vi "CALC_Calculate_phi_theta_etc_2_(offline).vi"(0 "Input data cluster":T2, 1 "SB size":u8, 5 "Twisted neck":bool, 7 "Bridge swap":bool, 9 "Use alternative magnets orientation":bool, 11 "Error In":errorcluster) -> (4 "Animal coordinates cluster":T1, 15 "Error out":errorcluster)   [LabVIEW 2018, in "Tracker.lvlib"]
uses:
  Tracker.lvlib
  Controls/CTL_Cage_Coords_(arrays).ctl
  Controls/CTL_Animal_Coordinates_and_Speed_(arr).ctl
  Controls/CTL_Animal_Coordinates_and_Speed.ctl
  <vilib>/ptbypt/NI_PtbyPt.lvlib
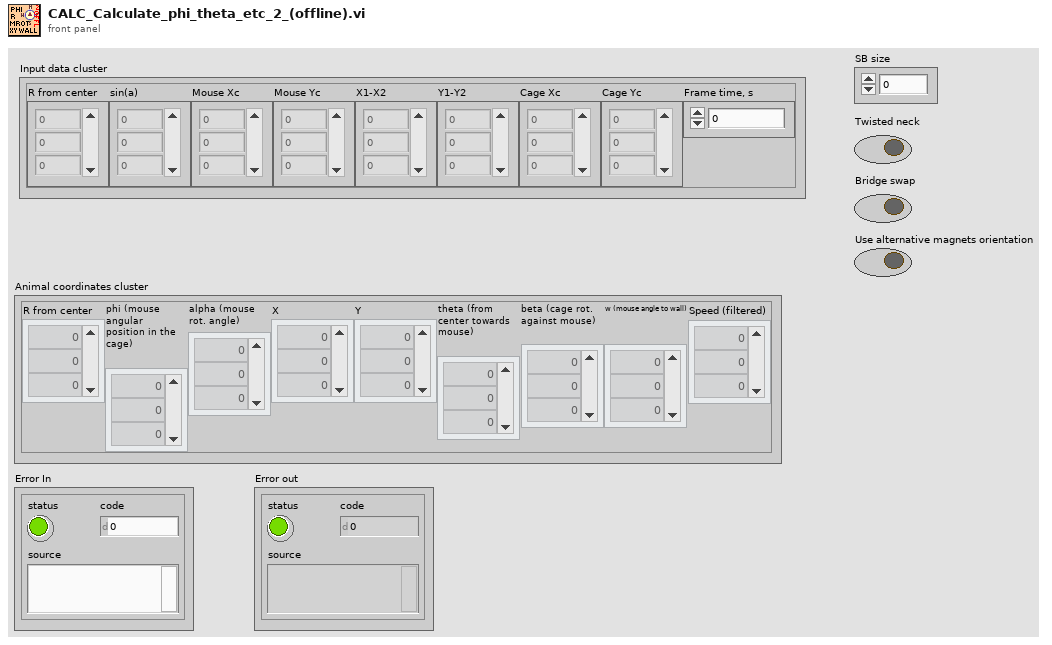
[diagram p1: front panel]
types:
  T1 = typedef "Tracker.lvlib/CTL_Animal_Coordinates_and_Speed_(arr).ctl" = cluster{"R from center":dbl[], "phi (mouse angular position in the cage)":dbl[], "alpha (mouse rot. angle)":dbl[], "X":dbl[], "Y":dbl[], "theta (from center towards mouse)":dbl[], "beta (cage rot. against mouse)":dbl[], "w (mouse angle to wall)":dbl[], "Speed (filtered)":dbl[]}
  T2 = typedef "Tracker.lvlib/CTL_Cage_Coords_(arrays).ctl" = cluster{"R from center":dbl[], "sin(a)":dbl[], "Mouse Xc":dbl[], "Mouse Yc":dbl[], "X1-X2":dbl[], "Y1-Y2":dbl[], "Cage Xc":dbl[], "Cage Yc":dbl[], "Frame time, s":dbl}
  T3 = typedef "Tracker.lvlib/CTL_Animal_Coordinates_and_Speed.ctl" = cluster{"R from center":dbl, "phi (mouse angular position in the cage)":dbl, "alpha (mouse rot. angle)":dbl, "X":dbl, "Y":dbl, "theta (from center towards mouse)":dbl, "beta (cage rot. against mouse)":dbl, "w (mouse angle to wall)":dbl, "Speed (filtered)":dbl}
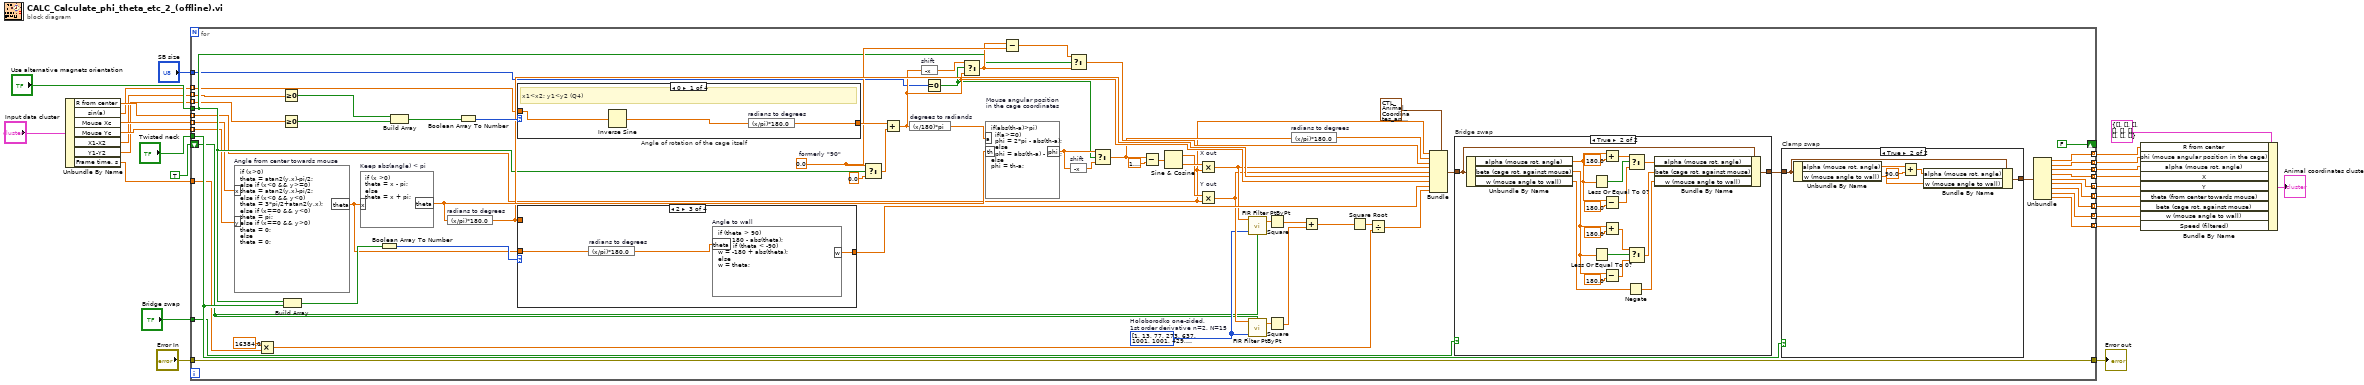
[diagram p0: block diagram]
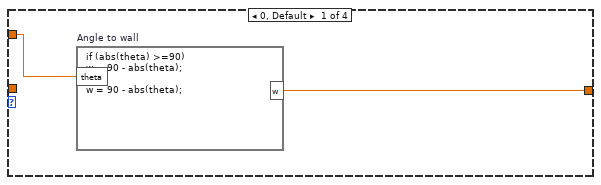
[diagram p3: hidden frame]
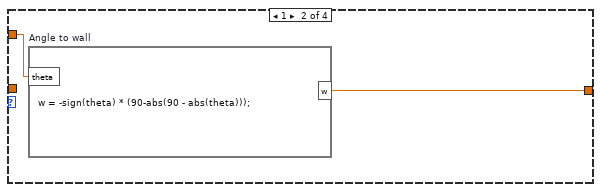
[diagram p4: hidden frame]
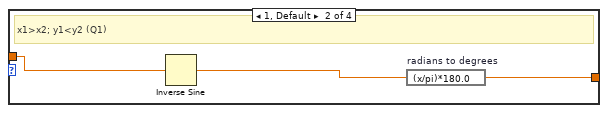
[diagram p7: hidden frame]
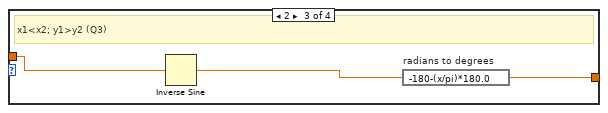
[diagram p8: hidden frame]
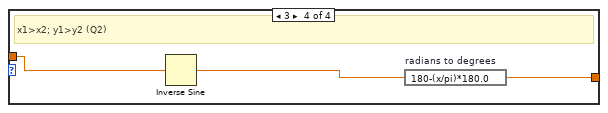
[diagram p9: hidden frame]
diagram:
  n1 = Unbundle By Name("Input data cluster") -> ("R from center"=w22:dbl[], "sin(a)"=w21:dbl[], "Mouse Xc"=w20:dbl[], "Mouse Yc"=w19:dbl[], "X1-X2"=w18:dbl[], "Y1-Y2"=w17:dbl[], "Frame time, s"=w16:dbl)
  n2 = for {
    tunnel: "Use alternative magnets orientation" -> [w67]
    tunnel: "Twisted neck" -> [w66]
    tunnel: "SB size" -> [w62]
    tunnel: "Bridge swap" -> [w48]
    tunnel: w22 -> [w47] mode=indexing
    tunnel: w21 -> [w46] mode=indexing
    tunnel: w20 -> [w45] mode=indexing
    tunnel: w19 -> [w44] mode=indexing
    tunnel: w18 -> [w43] mode=indexing
    tunnel: w17 -> [w42] mode=indexing
    tunnel: w16 -> [w41]
    tunnel: [w39] -> w13 mode=indexing
    tunnel: [w38] -> w12 mode=indexing
    tunnel: [w37] -> w11 mode=indexing
    tunnel: [w36] -> w10 mode=indexing
    tunnel: [w35] -> w9 mode=indexing
    tunnel: [w34] -> w8 mode=indexing
    tunnel: [w33] -> w7 mode=indexing
    tunnel: [w32] -> w6 mode=indexing
    tunnel: [w31] -> w5 mode=indexing
    tunnel: "Error In" -> [w30]
    tunnel: [w30] -> w2
    shift-right: [FALSE] -> _
    shift-left: TRUE -> [w29]
    w58 = i32[] [1, 13, 77, 273, 637, 1001, 1001, 429, -429, -1001, -1001, -637, -273, -77, -13, -1]  # Holoborodko one-sided, 1st order derivative n=2, N=15
    w77 = 0.0  # formerly "90"
    n3 = formula code="if (x>0)\ntheta = atan2(y,x)-pi/2;\nelse if (x<0 && y>=0)\ntheta = atan2(y,x)-pi/2;\nelse if (x<0 && y<0)\ntheta = 3*pi/2+atan2(y,x);\nelse if (x==0 && y<0)\ntheta = pi;\nelse if (x==0 && y>0)\ntheta = 0;\nelse\ntheta = 0;" "Angle from center towards mouse"("x"=w45, "y"=w44) -> ("theta"=w63:dbl)
    n4 = Multiply(x=16384.0 ("y"), y=w41) -> (x*y=w49:dbl)
    n5 = Greater Or Equal To 0?(x=w43) -> (x >= 0?=w94:bool)
    n6 = Greater Or Equal To 0?(x=w42) -> (x >= 0?=w93:bool)
    n7 = Build Array(w67, w66) -> (w65:bool[])
    n8 = formula code="if (x >0)\ntheta = x - pi;\nelse\ntheta = x + pi;" "Keep abs(angle) < pi"("x"=w63) -> ("theta"=w88:dbl)
    n9 = Boolean Array To Number(Boolean array=w65) -> (number=w64:u32)
    n10 = Build Array(w94, w93) -> (w92:bool[])
    n11 = expression code="(x/pi)*180.0" "radians to degrees"(w88) -> (w84:dbl)
    n12 = Boolean Array To Number(Boolean array=w92) -> (number=w91:u32)
    n13 = case "Angle of rotation of the cage itself" shown="0" w91 {
      tunnel: w46 -> [w130 w133 w136 w139]
      tunnel: [w129 w132 w135 w138] -> w80
      frame 0 {
        # "x1<x2; y1<y2 (Q4)"
        n14 = Inverse Sine(1:w130) -> (0:w131:dbl)
        n15 = expression code="(x/pi)*180.0" "radians to degrees"(w131) -> (w129:dbl)
      }
      frame 1, Default {
        # "x1>x2; y1<y2 (Q1)"
        n16 = Inverse Sine(1:w133) -> (0:w134:dbl)
        n17 = expression code="(x/pi)*180.0" "radians to degrees"(w134) -> (w132:dbl)
      }
      frame 2 {
        # "x1<x2; y1>y2 (Q3)"
        n18 = Inverse Sine(1:w136) -> (0:w137:dbl)
        n19 = expression code="-180-(x/pi)*180.0" "radians to degrees"(w137) -> (w135:dbl)
      }
      frame 3 {
        # "x1>x2; y1>y2 (Q2)"
        n20 = Inverse Sine(1:w139) -> (0:w140:dbl)
        n21 = expression code="180-(x/pi)*180.0" "radians to degrees"(w140) -> (w138:dbl)
      }
    }
    n22 = case shown="2" w64 {
      tunnel: w84 -> [w103 w105 _ w109]
      tunnel: [w102 w104 w108 w109] -> w68
      tunnel: w63 -> [_ _ w107 _]
      frame 0, Default {
        n23 = formula code="if (abs(theta) >=90)\nw = 90 - abs(theta);\nelse\nw = 90 - abs(theta);" "Angle to wall"("theta"=w103) -> ("w"=w102:dbl)
      }
      frame 1 {
        n24 = formula code="w = -sign(theta) * (90-abs(90 - abs(theta)));" "Angle to wall"("theta"=w105) -> ("w"=w104:dbl)
      }
      frame 2 {
        n25 = expression code="(x/pi)*180.0" "radians to degrees"(w107) -> (w106:dbl)
        n26 = formula code="if (theta > 90)\nw = 180 - abs(theta);\nelse if (theta < -90)\nw = -180 + abs(theta);\nelse\nw = theta;" "Angle to wall"("theta"=w106) -> ("w"=w108:dbl)
      }
      frame 3 {
      }
    }
    n27 = Select(t=w77, s=w67, f=0.0) -> (s? t:f=w76:dbl)
    n28 = Add(x=w80, y=w76) -> (x+y=w74:dbl)
    n29 = expression code="(x/180)*pi" "degrees to radiands"(w74) -> (w87:dbl)
    n30 = expression code="-x" "shift"(w74) -> (w73:dbl)
    n31 = Equal To 0?(x=w62) -> (x = 0?=w61:bool)
    n32 = Select(t=w73, s=w61, f=w74) -> (s? t:f=w75:dbl)
    n33 = formula code="if(abs(th-a)>pi)\n  if(a>=0)\n  phi = 2*pi - abs(th-a);\n  else\n  phi = abs(th-a) - 2*pi;\nelse\nphi = th-a;" "Mouse angular position in the cage coordinates"("th"=w88, "a"=w87) -> ("phi"=w71:dbl)
    n34 = Subtract(x=w75, y=w77) -> (x-y=w78:dbl)
    n35 = Select(t=w78, s=w67, f=w75) -> (s? t:f=w79:dbl)
    n36 = expression code="-x" "shift"(w71) -> (w70:dbl)
    n37 = Select(t=w71, s=w61, f=w70) -> (s? t:f=w72:dbl)
    n38 = Subtract(x=w72, y=1.5707963267948966) -> (x-y=w86:dbl)
    n39 = Sine & Cosine(0:w86) -> (1:w89:dbl, 2:w90:dbl)
    n40 = Multiply "X out"(x=w90, y=w47) -> (x*y=w60:dbl)
    n41 = Multiply "Y out"(x=w89, y=w47) -> (x*y=w59:dbl)
    n42 = call <vilib>:"FIR Filter PtByPt.vi"("initialize"=w29, "Forward Coefficients"=w58, "x"=w60) -> ("Filtered x"=w57:dbl)  [unwired: 1 in, 1 out]
    n43 = call <vilib>:"FIR Filter PtByPt.vi"("initialize"=w29, "Forward Coefficients"=w58, "x"=w59) -> ("Filtered x"=w56:dbl)  [unwired: 1 in, 1 out]
    n44 = Square(x=w57) -> (x^2=w55:dbl)
    n45 = Square(x=w56) -> (x^2=w54:dbl)
    n46 = expression code="(x/pi)*180.0" "radians to degrees"(w72) -> (w83:dbl)
    n47 = Add(x=w55, y=w54) -> (x+y=w53:dbl)
    n48 = Square Root(x=w53) -> (sqrt(x)=w50:dbl)
    n49 = Divide(x=w50, y=w49) -> (x/y=w52:dbl)
    n50 = Bundle(cluster=T3 {"R from center"=0.0, "phi (mouse angular position in the cage)"=0.0, "alpha (mouse rot. angle)"=0.0, "X"=0.0, "Y"=0.0, "theta (from center towards mouse)"=0.0, "beta (cage rot. against mouse)"=0.0, "w (mouse angle to wall)"=0.0, "Speed (filtered)"=0.0} ("Animal coordinates and speed"), "R from center"=w47, "phi (mouse angular position in the cage)"=w83, "alpha (mouse rot. angle)"=w79, "X"=w60, "Y"=w59, "theta (from center towards mouse)"=w84, "beta (cage rot. against mouse)"=w74, "w (mouse angle to wall)"=w68, "Speed (filtered)"=w52) -> (w82:T3)
    n51 = case "Bridge swap" shown="True" w48 {
      tunnel: [w110 w122] -> w69
      tunnel: w82 -> [w110 w123]
      frame False {
      }
      frame True {
        n52 = Unbundle By Name(w123) -> ("alpha (mouse rot. angle)"=w121:dbl, "beta (cage rot. against mouse)"=w114:dbl, "w (mouse angle to wall)"=w112:dbl)
        n53 = Less Or Equal To 0?(x=w121) -> (x <= 0?=w128:bool)
        n54 = Less Or Equal To 0?(x=w114) -> (x <= 0?=w115:bool)
        n55 = Add(x=w121, y=sgl 180.0) -> (x+y=w125:dbl)
        n56 = Subtract(x=w121, y=sgl 180.0) -> (x-y=w127:dbl)
        n57 = Add(x=w114, y=sgl 180.0) -> (x+y=w118:dbl)
        n58 = Subtract(x=w114, y=sgl 180.0) -> (x-y=w116:dbl)
        n59 = Negate(x=w112) -> (-x=w111:dbl)
        n60 = Select(t=w125, s=w128, f=w127) -> (s? t:f=w120:dbl)
        n61 = Select(t=w118, s=w115, f=w116) -> (s? t:f=w113:dbl)
        n62 = Bundle By Name(cluster=w123, "alpha (mouse rot. angle)"=w120, "beta (cage rot. against mouse)"=w113, "w (mouse angle to wall)"=w111) -> (w122:T3)
      }
    }
    n63 = case "Clamp swap" shown="True" w66 {
      tunnel: [w95 w99] -> w40
      tunnel: w69 -> [w95 w100]
      frame False {
      }
      frame True {
        n64 = Unbundle By Name(w100) -> ("alpha (mouse rot. angle)"=w98:dbl, "w (mouse angle to wall)"=w97:dbl)
        n65 = Add(x=w98, y=sgl 90.0) -> (x+y=w96:dbl)
        n66 = Bundle By Name(cluster=w100, "alpha (mouse rot. angle)"=w96, "w (mouse angle to wall)"=w97) -> (w99:T3)
      }
    }
    n67 = Unbundle(w40) -> ("R from center"=w39:dbl, "phi (mouse angular position in the cage)"=w38:dbl, "alpha (mouse rot. angle)"=w37:dbl, "X"=w36:dbl, "Y"=w35:dbl, "theta (from center towards mouse)"=w34:dbl, "beta (cage rot. against mouse)"=w33:dbl, "w (mouse angle to wall)"=w32:dbl, "Speed (filtered)"=w31:dbl)
  }
  "Error out" <- w2
  n68 = Bundle By Name(cluster=T1 {"R from center"=[], "phi (mouse angular position in the cage)"=[], "alpha (mouse rot. angle)"=[], "X"=[], "Y"=[], "theta (from center towards mouse)"=[], "beta (cage rot. against mouse)"=[], "w (mouse angle to wall)"=[], "Speed (filtered)"=[]} ("Animal coordinates and speed"), "R from center"=w13, "phi (mouse angular position in the cage)"=w12, "alpha (mouse rot. angle)"=w11, "X"=w10, "Y"=w9, "theta (from center towards mouse)"=w8, "beta (cage rot. against mouse)"=w7, "w (mouse angle to wall)"=w6, "Speed (filtered)"=w5) -> (→"Animal coordinates cluster":T1)
